vi "ranges_config_get_double.vi"(4 "key":string) -> (1 "value":dbl, 2 "found?":bool)   [LabVIEW 2017]
uses:
  <vilib>/Utility/config.llb/Read Key (Double).vi
  <vilib>/Utility/config.llb/NI_LVConfig.lvlib
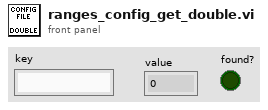
[diagram p1: front panel]
types:
  T1 = typedef "NI_LVConfig.lvlib/Config Data RefNum.ctl" = refnum<k1>
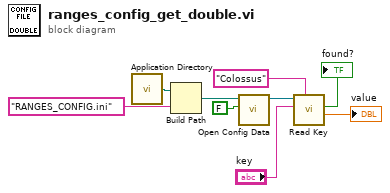
[diagram p0: block diagram]
diagram:
  n1 = call <vilib>:"Application Directory.vi"() -> ("Application Directory"=w6:path)
  n2 = Build Path(base path=w6, name or relative path="RANGES_CONFIG.ini") -> (appended path=w7:path)
  n3 = call <vilib>:"Open Config Data.vi"("create file if necessary (T)"=FALSE, "configuration file path"=w7) -> ("refnum"=w5:T1)  [unwired: 7 in, 2 out]
  n4 = call-poly <vilib>:"Read Key.vi"("section"="Colossus", "key"="key", "refnum"=w5) -> ("value"=→"value":dbl, "found?"=→"found?":bool)  [unwired: 5 in, 2 out]
